vi "Main Page.vi"(8 "error in (no error)":errorcluster, 11 "Node Ptr":T1 format="%.0x") -> (0 "error out":errorcluster)   [LabVIEW 2015, in "DDS Custom Device System Explorer.lvlib"]
uses:
  DDS Custom Device System Explorer.lvlib
  <vilib>/NI Veristand/Custom Device API/Custom Device Item Ref.ctl
  <vilib>/NI VeriStand/Custom Device API/Custom Device API.lvlib
panel:
  out "Version":string
  in  "SHDocVw.IWebBrowser":refnum<k7>(container)
  in  "Specific Header":cluster{"Section Name":string}={"Section Name"="Custom Device Item Settings"}
  in  "General Header":cluster{"Section Name":string}={"Section Name"="General Custom Device Settings"}
  in  "Description":string
  in  "Name":string
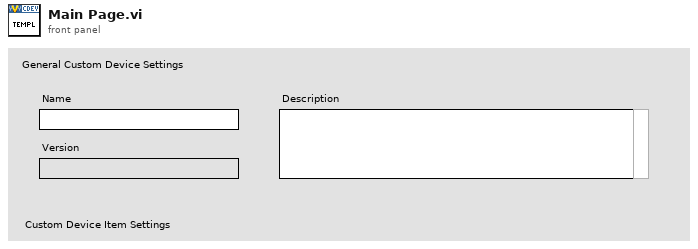
[diagram p1: front panel]
types:
  T1 = typedef "Custom Device API.lvlib/Custom Device Item Ref.ctl" = u64
  T2 = typedef "Custom Device API.lvlib/Custom Device Item Info.ctl" = cluster{"Name":string, "Is Channel":bool, "GUID":string, "Is Waveform":bool}
  T3 = typedef "Custom Device API.lvlib/Custom Device Commands.ctl" = enum16{"Default", "Item renamed", "Shutdown", "Dynamic button pressed"}
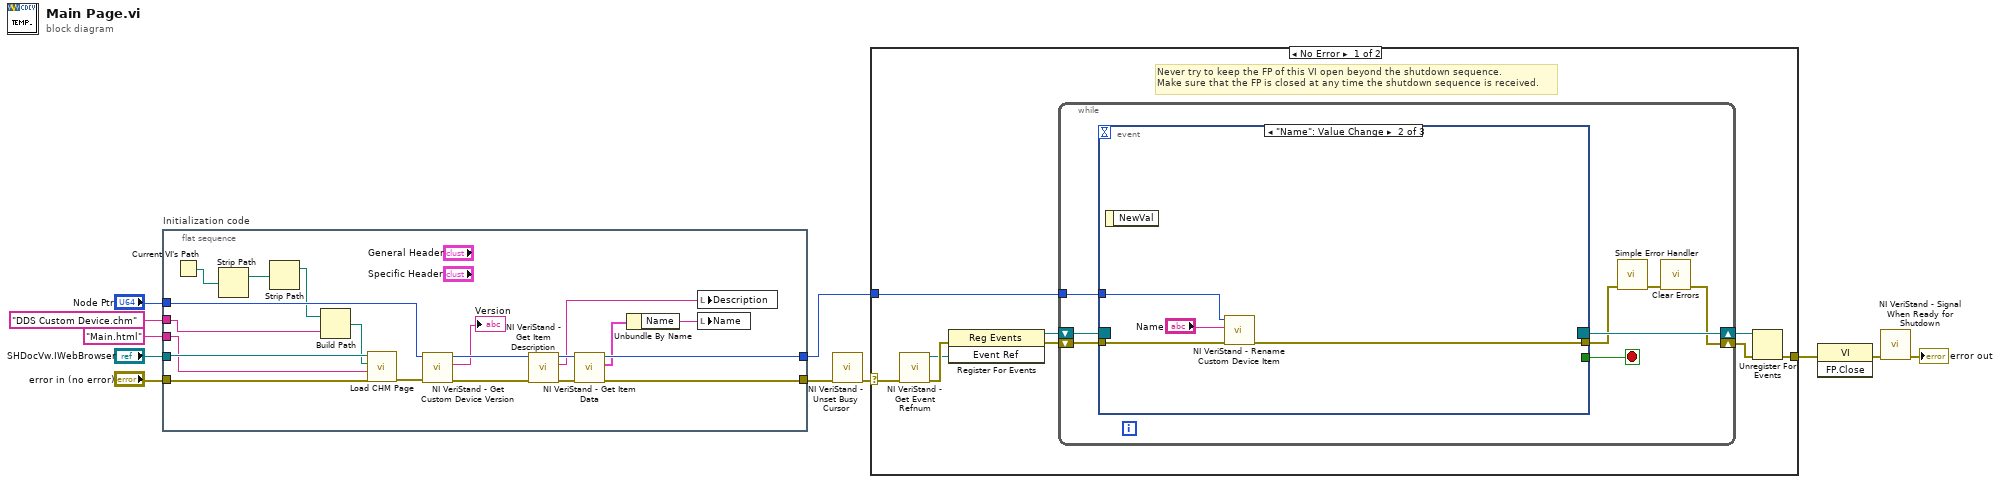
[diagram p0: block diagram]
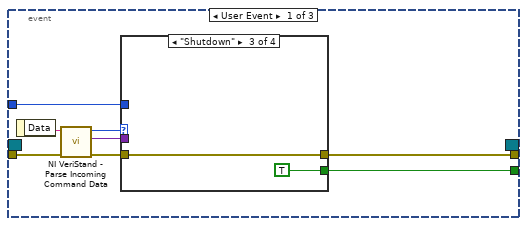
[diagram p2: hidden frame]
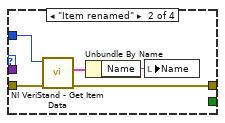
[diagram p4: hidden frame]
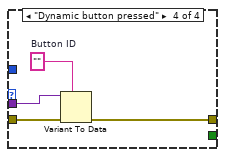
[diagram p5: hidden frame]
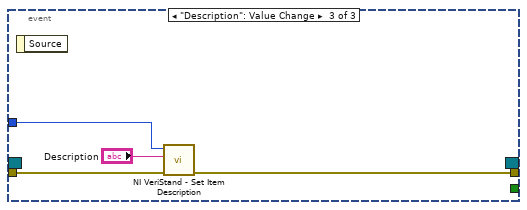
[diagram p6: hidden frame]
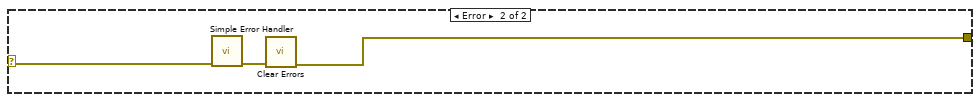
[diagram p7: hidden frame]
diagram:
  n1 = flat-sequence "Initialization code" {
    tunnel: "error in (no error)" -> [w15]
    tunnel: "Node Ptr" -> [w26]
    tunnel: [w27] -> w7
    tunnel: [w31] -> w4
    tunnel: "SHDocVw.IWebBrowser" -> [w16]
    tunnel: "Main.html" ("HTML File") -> [w12]
    tunnel: "DDS Custom Device.chm" ("CD_CHM_FileName") -> [w17]
    frame #0 {
      n2 = Current VI's Path() -> (path=w20:path)
      n3 = Strip Path(path=w20) -> (stripped path=w19:path)  [unwired: 1 out]
      n4 = Strip Path(path=w19) -> (stripped path=w18:path)  [unwired: 1 out]
      n5 = Build Path(base path=w18, name or relative path=w17) -> (appended path=w13:path)
      n6 = call <vilib>:"Load CHM Page.vi"("error in (no error)"=w15, "HTML File"=w12, "Main CHM File Path"=w13, "Web Browser Reference"=w16) -> ("error out"=w14:errorcluster)  [unwired: 7 in]
      n7 = call <vilib>:"NI VeriStand - Get Custom Device Version.vi"("error in (no error)"=w14, "Device Ref in"=w26) -> ("error out"=w25:errorcluster, "Value"=→"Version":string, "Device Ref out"=w24:T1)  [unwired: 7 in]
      n8 = call <vilib>:"NI VeriStand - Get Item Description.vi"("error in (no error)"=w25, "Item Ref in"=w24) -> ("error out"=w29:errorcluster, "Description"=w21:string, "Item Ref out"=w30:T1)  [unwired: 7 out]
      n9 = call <vilib>:"NI VeriStand - Get Item Data.vi"("error in (no error)"=w29, "Item Ref in"=w30) -> ("error out"=w27:errorcluster, "Item Info"=w28:T2, "Item Ref out"=w31:T1)  [unwired: 7 out]
      n10 = Unbundle By Name(w28) -> ("Name"=w22:string)
      n11 = local write "Description"(w21) -> ()
      n12 = local write "Name"(w22) -> ()
    }
  }
  n13 = call <vilib>:"NI VeriStand - Unset Busy Cursor.vi"("error in (no error)"=w7) -> ("error out"=w6:errorcluster)  [unwired: 10 out]
  n14 = case shown="No Error" w6 {
    selector: w6 -> [w32 w79]
    tunnel: [w37 w77] -> w11
    tunnel: w4 -> [w33 _]
    frame No Error {
      # "Never try to keep the FP of this VI open beyond the shutdown sequence.\nMake sure that the FP is closed at any time the shutdown sequence is received."
      n15 = call <vilib>:"NI VeriStand - Get Event Refnum.vi"("error in (no error)"=w32) -> ("error out"=w40:errorcluster, "Event Ref"=w36:refnum<user-event>)  [unwired: 9 out]
      n16 = register-events(error in=w40, w36) -> (reference out=w34:refnum<event-registration>, error out=w35:errorcluster)  [unwired: 1 in]
      n17 = while {
        tunnel: w33 -> [w44]
        shift-right: [w41] -> w38
        shift-left: w35 -> [w47]
        shift-right: [w48] -> w39
        shift-left: w34 -> [w46]
        stop <- w45 stop-if-true
        n18 = event shown="[1] \"Name\": Value Change" {
          selector: w46 -> [_ _ _]
          dyn-events: [_ _ _] -> w48
          timeout: _ -> [_ _ _]
          tunnel: w47 -> [w56 w72 w75]
          tunnel: [w52 _ _] -> w45
          tunnel: [w51 w71 w74] -> w43
          tunnel: w44 -> [w50 w70 w76]
          event User Event {
            n19 = event-data() -> ("Data"=w55:string)  [unwired: 1 out]
            n20 = call <vilib>:"NI VeriStand - Parse Incoming Command Data.vi"("error in (no error)"=w56, "Incoming data"=w55) -> ("error out"=w54:errorcluster, "Outgoing data"=w49:variant, "Action"=w53:T3)  [unwired: 7 out]
            n21 = case shown="\"Shutdown\"" w53 {
              tunnel: w54 -> [w57 w62 w63 w68]
              tunnel: [_ _ TRUE _] -> w52
              tunnel: [w57 w59 w63 w65] -> w51
              tunnel: w50 -> [_ w61 _ _]
              tunnel: w49 -> [_ _ _ w67]
              frame "Default", Default {
              }
              frame "Item renamed" {
                n22 = call <vilib>:"NI VeriStand - Get Item Data.vi"("error in (no error)"=w62, "Item Ref in"=w61) -> ("error out"=w59:errorcluster, "Item Info"=w60:T2)  [unwired: 8 out]
                n23 = Unbundle By Name(w60) -> ("Name"=w58:string)
                n24 = local write "Name"(w58) -> ()
              }
              frame "Shutdown" {
              }
              frame "Dynamic button pressed" {
                w66 = ""  # Button ID
                n25 = Variant To Data(error in=w68, type=w66, Variant=w67) -> (error out=w65:errorcluster)  [unwired: 1 out]
              }
            }
          }
          event "Name": Value Change {
            n26 = event-data() -> ()  [unwired: 2 out]
            n27 = call <vilib>:"NI VeriStand - Rename Custom Device Item.vi"("error in (no error)"=w72, "New Name"="Name", "Item Ref in"=w70) -> ("error out"=w71:errorcluster)  [unwired: 1 in, 7 out]
          }
          event "Description": Value Change {
            n28 = event-data() -> ()  [unwired: 2 out]
            n29 = call <vilib>:"NI VeriStand - Set Item Description.vi"("error in (no error)"=w75, "Description"="Description", "Item Ref in"=w76) -> ("error out"=w74:errorcluster)  [unwired: 8 out]
          }
        }
        n30 = call <vilib>:"Simple Error Handler.vi"("error in (no error)"=w43) -> ("error out"=w42:errorcluster)  [unwired: 1 in, 7 out]
        n31 = call <vilib>:"Clear Errors.vi"("error in (no error)"=w42) -> ("error out"=w41:errorcluster)  [unwired: 1 in, 5 out]
      }
      n32 = Unregister For Events(event registration refnum=w39, error in=w38) -> (error out=w37:errorcluster)
    }
    frame Error {
      n33 = call <vilib>:"Simple Error Handler.vi"("error in (no error)"=w79) -> ("error out"=w78:errorcluster)  [unwired: 1 in, 7 out]
      n34 = call <vilib>:"Clear Errors.vi"("error in (no error)"=w78) -> ("error out"=w77:errorcluster)  [unwired: 1 in, 5 out]
    }
  }
  n35 = invoke class="VI" method="FP.Close"(error in=w11) -> (error out=w10:errorcluster)  [unwired: 2 in, 2 out]
  n36 = call <vilib>:"NI VeriStand - Signal When Ready for Shutdown.vi"("error in (no error)"=w10) -> ("error out"=→"error out":errorcluster)  [unwired: 10 out]
